vi "AI channel settings.vi"(8 "error in (no error)":errorcluster, 11 "Refnum in":refnum<k21>) -> (0 "error out":errorcluster, 3 "Refnum out":refnum<k21>)   [LabVIEW 2018]
uses:
  AI channel settings.ctl
  <vilib>/DAQmx/create/channels.llb/DAQmx Create Channel (AI-Voltage-Basic).vi
panel:
  out "AI channel settings out":T1 {"units" items=["Volts"=10348, "From TEDS"=12516, "From Custom Scale"=10065]}
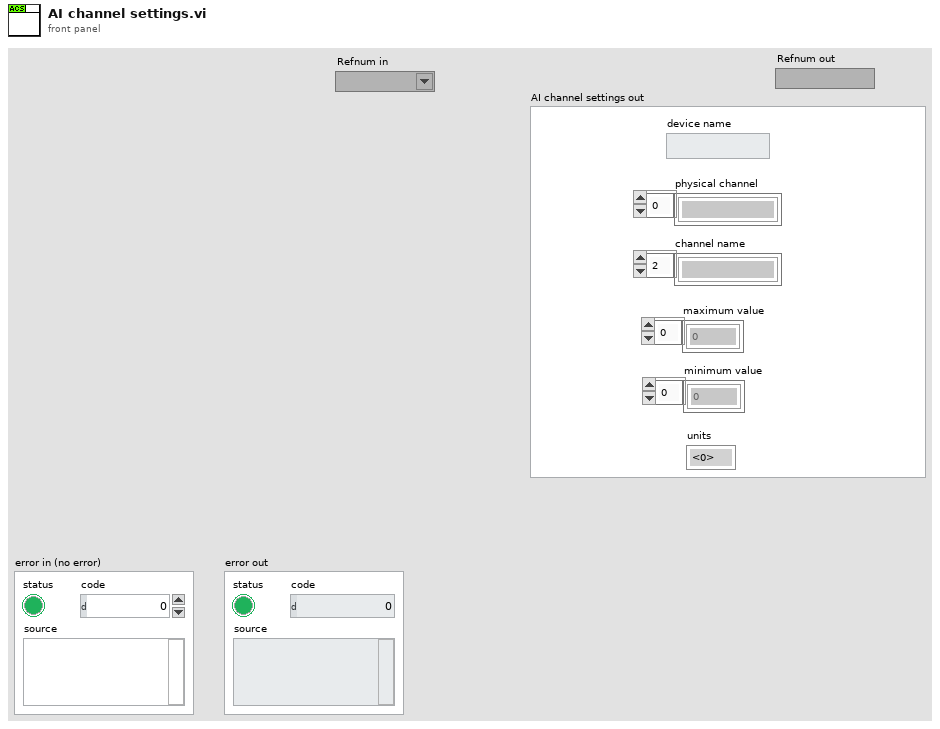
[diagram p1: front panel]
types:
  T1 = typedef "AI channel settings.ctl" = cluster{"device name":string, "physical channel":string[], "channel name":string[], "maximum value":dbl[], "minimum value":dbl[], "units":i32}
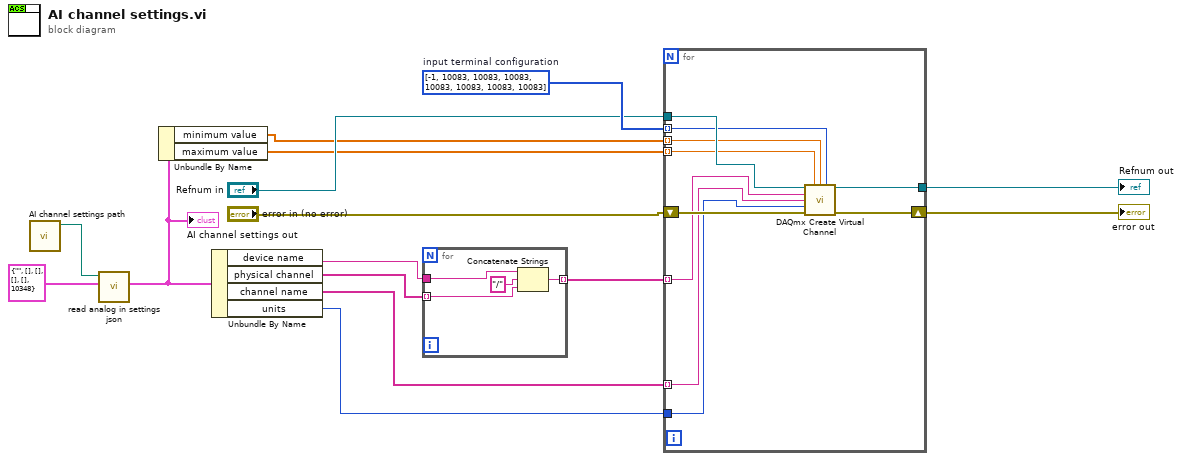
[diagram p0: block diagram]
diagram:
  w12 = i32[] [-1, 10083, 10083, 10083, 10083, 10083, 10083, 10083] items=["default"=-1, "RSE"=10083, "NRSE"=10078, "Differential"=10106, "Pseudodifferential"=12529]  # input terminal configuration
  n1 = call "AI channel settings path.vi"() -> ("appended path"=w1:path)  [unwired: 11 in]
  n2 = call "read analog in settings json.vi"("AI channel type"=T1 {"device name"="", "physical channel"=[], "channel name"=[], "maximum value"=[], "minimum value"=[], "units"=10348} ("AI channel settings"), "appended path"=w1) -> ("AI channel settings out"=w2:T1)  [unwired: 9 in]
  "AI channel settings out" <- w2
  n3 = Unbundle By Name(w2) -> ("minimum value"=w5:dbl[], "maximum value"=w4:dbl[])
  n4 = Unbundle By Name(w2) -> ("device name"=w9:string, "physical channel"=w8:string[], "channel name"=w7:string[], "units"=w6:i32)
  n5 = for {
    tunnel: [w19] -> w13 mode=indexing
    tunnel: w9 -> [w18]
    tunnel: w8 -> [w16] mode=indexing
    n6 = Concatenate Strings(w18, "/" ("string"), w16) -> (w19:string)
  }
  n7 = for {
    tunnel: "Refnum in" -> [w29]
    tunnel: [w27] -> w14
    tunnel: w12 -> [w25] mode=indexing
    tunnel: w5 -> [w24] mode=indexing
    tunnel: w4 -> [w23] mode=indexing
    tunnel: w13 -> [w22] mode=indexing
    tunnel: w7 -> [w21] mode=indexing
    tunnel: w6 -> [w20]
    shift-right: [w26] -> w15
    shift-left: "error in (no error)" -> [w28]
    n8 = call-poly <vilib>:"DAQmx Create Virtual Channel.vi"("task in"=w29, "maximum value"=w23, "minimum value"=w24, "input terminal configuration"=w25, "physical channels"=w22, "name to assign"=w21, "units"=w20, "error in"=w28) -> ("task out"=w27:refnum<k21>, "error out"=w26:errorcluster)  [unwired: 6 in]
  }
  "error out" <- w15
  "Refnum out" <- w14
